vi "ITC Reply to PGSQL.vi"(8 "error in (no error)":errorcluster, 10 "Response":T1, 11 "Instrument.1820 in":refnum<class "Instrument.OxfordVRM.lvclass">) -> (0 "error out":errorcluster, 3 "Instrument.1820 out":refnum<class "Instrument.OxfordVRM.lvclass">)   [LabVIEW 2016, in "Instrument.OxfordVRM.lvclass"]
uses:
  Instrument.OxfordVRM.lvclass
  <instrlib>/Mercury iXX/Public/Controls/Response String.ctl
  <userlib>/LevyLab/Levylab Instruments/SMOs/Logger.PGSQL/Logger.PGSQL.lvclass
  <userlib>/LevyLab/Levylab Instruments/SMOs/Instrument/Instrument.lvclass
  C:/Program Files (x86)/National Instruments/LabVIEW 2016/user.lib/LevyLab/Levylab Instruments/SMOs/Instrument/Instrument.lvclass
  <instrlib>/Mercury iXX/Mercury iXX.lvlib
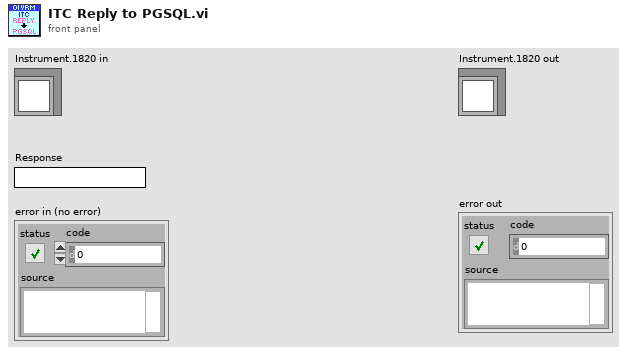
[diagram p1: front panel]
types:
  T1 = typedef "Mercury iXX.lvlib/Response String.ctl" = string
  T2 = typedef "Instrument.lvclass/Dependencies--Cluster.ctl" = cluster{"RemoteControl":refnum<class "RemoteControl.lvclass">, "Logger.Error":refnum<class "Logger.Error.lvclass">, "Logger.PGSQL":refnum<class "Logger.PGSQL.lvclass">}
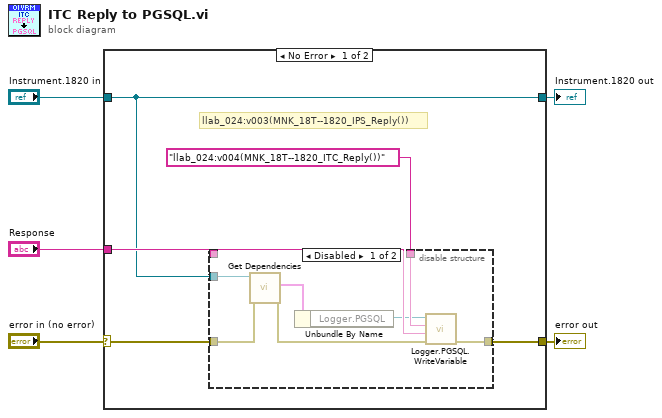
[diagram p0: block diagram]
diagram:
  n1 = case shown="No Error" "error in (no error)" {
    selector: "error in (no error)" -> [w7 w19]
    tunnel: "Response" -> [w10 _]
    tunnel: [w8 w19] -> w4
    tunnel: "Instrument.1820 in" -> [w6 w20]
    tunnel: [w6 w20] -> w1
    frame No Error {
      # "llab_024:v003(MNK_18T--1820_IPS_Reply())"
      n2 = disable-structure shown="Disabled" {
        disable-tunnel: w10 -> [w18 _]
        disable-tunnel: "llab_024:v004(MNK_18T--1820_ITC_Reply())" ("variable") -> [w17 _]
        disable-tunnel: [w16 _] -> w8
        disable-tunnel: w7 -> [w12 _]
        disable-tunnel: w6 -> [w11 _]
        frame Disabled {
          n3 = call <userlib>:"Get Dependencies.vi"("error in (no error)"=w12, "Instrument in"=w11) -> ("error out"=w13:errorcluster, "Dependencies"=w14:T2)  [unwired: 7 in, 1 out]
          n4 = Unbundle By Name(w14) -> ("Logger.PGSQL"=w15:refnum<class "Logger.PGSQL.lvclass">)
          n5 = call <userlib>:"Logger.PGSQL.WriteVariable.vi"("error in (no error)"=w13, "Data"=w18, "Address"=w17, "Logger"=w15) -> ("error out"=w16:errorcluster)  [unwired: 6 in, 1 out]
        }
        frame Enabled {
        }
      }
    }
    frame Error {
    }
  }
  "error out" <- w4
  "Instrument.1820 out" <- w1
